vi "sv_Get Nominal Frequency.vi"(8 "frequency range [Hz]":cluster{"low freq.":dbl, "high freq.":dbl}={"low freq."=1000.0, "high freq."=1000.0} {"high freq." min=0.001 format="%.2f"; "low freq." min=0.001 format="%.2f"}, 10 "octave info":T1={"standard"=enum."ANSI S1.11", "bandwidth"=enum."1 octave", "low band"=0, "high band"=0, "weighting filter"=0, "dB reference"=0.0, "dB On"=FALSE, "unit label"="", "channel name"="", "description"="", "engineering units"=1, "custom label"="", "spectrum type"=enum."magnitude", "spectral density"=FALSE, "filters settled"=FALSE} {"engineering units" items=["custom..."=0, "V"=1, "A"=21, "C"=30, "pC"=31, "s"=32, "-"=29, "Pa"=2, "N"=20, "g"=3, "m/s^2"=4, "m/s"=5, "m"=6, "mm/s"=12, "mm"=13, "micron/s"=14, "micron"=15, "in/s^2"=7, "in/s"=8, "in"=9, "mil/s"=10, "mil"=11, "rad/s^2"=16, "rad/s"=17, "rad"=18, "deg/s^2"=26, "deg/s"=27, "deg"=28, "RPM"=22, "cycle/s^2"=23, "Hz"=24, "cycle"=25, "strain"=19]; "dB reference" format="%.2e"; "weighting filter" items=["Linear", "A-weighting", "B-weighting", "C-weighting", "ITU-R 468-4", "Dolby", "CCITT", "C-message", "Wb", "Wc", "Wd", "We", "Wf", "Wh", "Wj", "Wk", "Wm", "AES17 20 kHz lowpass", "AES17 40 kHz lowpass", "AES17 20 kHz highpass", "AES17 40 kHz highpass"]}) -> (0 "high band":i32, 1 "low band":i32, 2 "high nominal frequency [Hz]":dbl, 3 "low nominal frequency [Hz]":dbl)   [LabVIEW 2017, in "SoundVib_Octave.lvlib"]
doc: "Takes the input <B>frequency range</B> and returns the low & high nominal frequencies as well as low & high bands that correspond to the input <B>frequency range</B>"
uses:
  <vilib>/addons/Sound and Vibration/svt_Octave/SoundVib_Octave.lvlib
  <vilib>/addons/_NISVFA/_Shared subVIs/Controls/svc_Octave Info.ctl
  <vilib>/addons/_NISVFA/_Shared subVIs/Controls/svc_Octave Standard.ctl
  <vilib>/addons/_NISVFA/_Shared subVIs/Controls/svc_Weighting Filter Text Ring.ctl
  <vilib>/addons/_NISVFA/_Shared subVIs/Controls/svc_Engineering Units Text Ring.ctl
  <vilib>/addons/Sound and Vibration/svt_Octave_2014 standard/SoundVib_Octave_2014 standard.lvlib
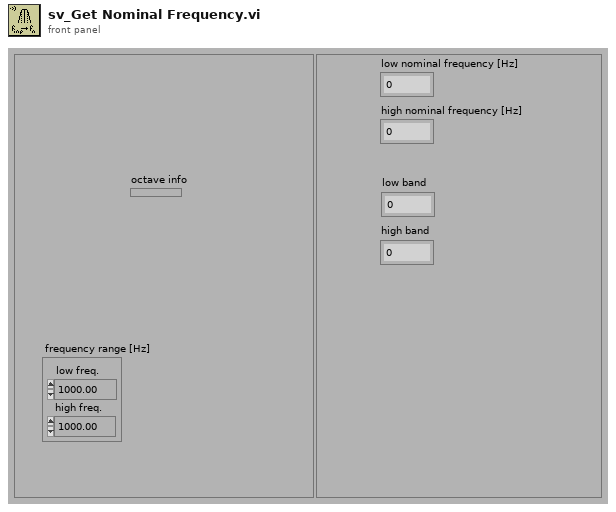
[diagram p1: front panel]
types:
  T1 = typedef "svc_Octave Info.ctl" = cluster{"standard":T2, "bandwidth":enum16{"1 octave", "1/3 octave", "1/6 octave", "1/12 octave", "1/24 octave"}, "low band":i32, "high band":i32, "weighting filter":T3, "dB reference":dbl, "dB On":bool, "unit label":string, "channel name":string, "description":string, "engineering units":T4, "custom label":string, "spectrum type":enum16{"power", "magnitude"}, "spectral density":bool, "filters settled":bool}
  T2 = typedef "svc_Octave Standard.ctl" = enum16{"ANSI S1.11", "IEC 61260"}
  T3 = typedef "svc_Weighting Filter Text Ring.ctl" = u16
  T4 = typedef "svc_Engineering Units Text Ring.ctl" = u16
  T5 = enum16{"1 octave", "1/3 octave", "1/6 octave", "1/12 octave", "1/24 octave"}
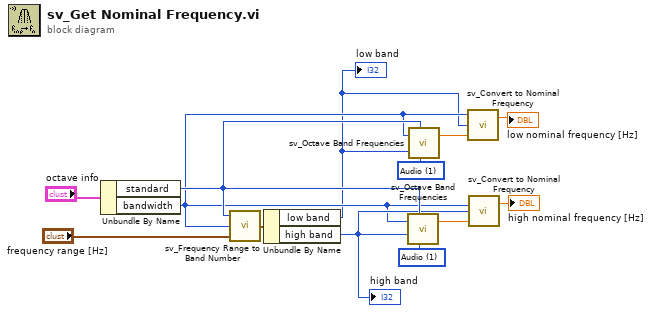
[diagram p0: block diagram]
diagram:
  w2 = u16 1 items=["Infrasonic", "Audio", "Ultrasonic"] ("Frequency range")
  w3 = u16 1 items=["Infrasonic", "Audio", "Ultrasonic"] ("Frequency range")
  n1 = Unbundle By Name("octave info") -> ("standard"=w6:T2, "bandwidth"=w4:T5)
  n2 = call <vilib>:"sv_Frequency Range to Band Number.vi"("frequency range [Hz]"="frequency range [Hz]", "bandwidth"=w4, "standard"=w6) -> ("band number"=w12:cluster{"low band":i32, "high band":i32})
  n3 = Unbundle By Name(w12) -> ("low band"=w1:i32, "high band"=w5:i32)
  "low band" <- w1
  "high band" <- w5
  n4 = call <vilib>:"sv_Octave Band Frequencies.vi"("octave band selector"=w5, "reference frequency range"=w2, "bandwidth"=w4, "standard"=w6) -> ("midband frequency [Hz]"=w9:dbl)  [unwired: 3 out]
  n5 = call <vilib>:"sv_Octave Band Frequencies.vi"("octave band selector"=w1, "reference frequency range"=w3, "bandwidth"=w4, "standard"=w6) -> ("midband frequency [Hz]"=w13:dbl)  [unwired: 3 out]
  n6 = call <vilib>:"sv_Convert to Nominal Frequency.vi"("bandwidth"=w4, "octave band selector"=w1, "midband frequency [Hz]"=w13) -> ("nominal frequency [Hz]"=→"low nominal frequency [Hz]":dbl)  [unwired: 2 in, 1 out]
  n7 = call <vilib>:"sv_Convert to Nominal Frequency.vi"("bandwidth"=w4, "octave band selector"=w5, "midband frequency [Hz]"=w9) -> ("nominal frequency [Hz]"=→"high nominal frequency [Hz]":dbl)  [unwired: 2 in, 1 out]
